vi "FindLineSubVI.vi"(0 "Image In":T1, 1 "Image Dst":T1, 7 "error in":errorcluster) -> (20 "Image Out":T1(plugin-control), 21 "Lines Calibrated (Shape Detection 1)":T2(array[cluster]) {"End Point"."Y" format="%.2f"; "End Point"."X" format="%.2f"; "Start Point"."Y" format="%.2f"; "Start Point"."X" format="%.2f"}, 27 "error out":errorcluster)   [LabVIEW 2011]
doc: "Creates, edits, and runs vision algorithms using NI Vision Assistant.\n\nWhen you place this Express VI on the block diagram, NI Vision Assistant launches. Create an algorithm using the Vision Assistant processing functions. After you create an algorithm, you can select the controls and indicators that you want to be able to programmatically set in LabVIEW. Double-click the Vision Assistant Express VI to edit the algorithm."
uses:
  <vilib>/vision/Image Controls.llb/IMAQ Image.ctl
  <vilib>/vision/NI_Vision_Development_Module.lvlib
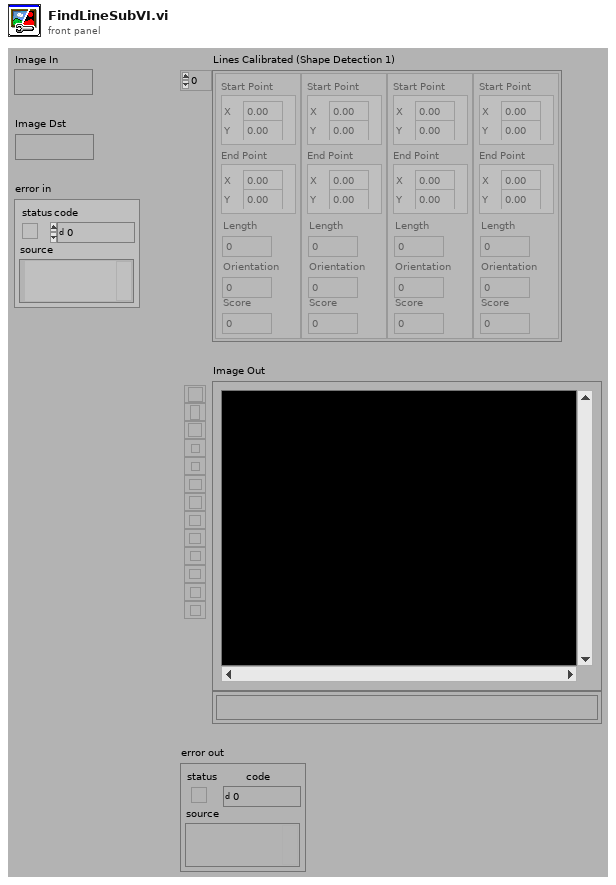
[diagram p1: front panel]
types:
  T1 = typedef "IMAQ Image.ctl" = refnum<image>
  T2 = cluster{"Start Point":cluster{"X":sgl, "Y":sgl}, "End Point":cluster{"X":sgl, "Y":sgl}, "Length":dbl, "Orientation":dbl, "Score":dbl}[]
  T3 = cluster{"Extraction Mode":u32, "Edge Threshold":i32, "Edge Filter Size":u32, "Min Length":i32, "Row Search Step Size":i32, "Col Search Step Size":i32, "Max Endpoint Gap":i32, "Closed":bool, "Subpixel":bool}
  T4 = cluster{"Rotation":bool, "Scale":bool, "Occlusion":bool, "Range Settings":cluster{"Match Constraints":u32, "Min":dbl, "Max":dbl}[]}
  T5 = cluster{"Global Rectangle":i32[], "Contours":cluster{"ID":enum32{"External", "Internal"}, "Type":u32, "Coordinates":i32[]}[]}
  T6 = typedef "Image Type" = u32
  T7 = cluster{"Start Point":cluster{"X":sgl, "Y":sgl}, "End Point":cluster{"X":sgl, "Y":sgl}, "Length":dbl, "Angle":dbl, "Score":dbl}[]
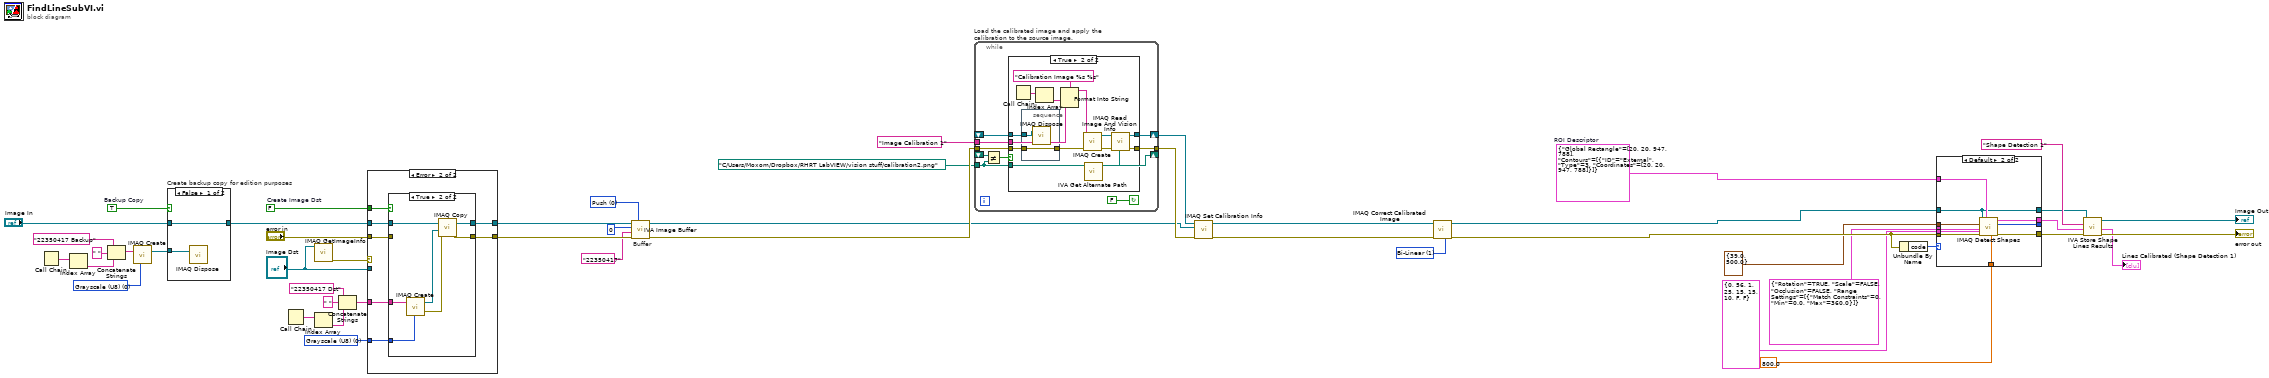
[diagram p0: block diagram]
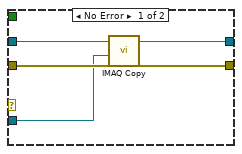
[diagram p4: hidden frame]
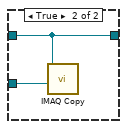
[diagram p6: hidden frame]
diagram:
  w10 = T5 {"Global Rectangle"=[20, 20, 947, 788], "Contours"=[{"ID"=enum."External", "Type"=3, "Coordinates"=[20, 20, 947, 788]}]}  # ROI Descriptor
  w17 = u32 1 items=["Zero Order", "Bi-Linear", "Quadratic", "Cubic Spline"] ("Interpolation Type")
  w26 = u16 0 items=["Push", "Pop", "Reset"] ("Function")
  w29 = T6 0 items=["Grayscale (U8)", "Grayscale (I16)", "Grayscale (SGL)", "Complex (CSG)", "RGB (U32)", "HSL (U32)", "RGB (U64)", "Grayscale (U16)"] ("Image Dst Type")
  w30 = T6 0 items=["Grayscale (U8)", "Grayscale (I16)", "Grayscale (SGL)", "Complex (CSG)", "RGB (U32)", "HSL (U32)", "RGB (U64)", "Grayscale (U16)"] ("Image Type")
  w49 = TRUE  # Backup Copy
  w42 = FALSE  # Create Image Dst
  # "Buffer"
  n1 = Call Chain() -> (call chain=w36:string[])
  n2 = Index Array(array=w36) -> (element=w35:string)  [unwired: 1 in]
  n3 = Concatenate Strings("22350417 Backup" ("Backup Image Name"), " ", w35) -> (w32:string)
  n4 = call "IMAQ Create"("Image Name"=w32, "Image Type"=w30) -> ("New Image"=w31:T1)  [unwired: 2 in, 2 out]
  n5 = case "Create backup copy for edition purposes" shown="False" w49 {
    tunnel: [w51 w53] -> w45
    tunnel: "Image In" -> [w51 w53]
    tunnel: w31 -> [w50 w52]
    frame False {
      n6 = call "IMAQ Dispose"("Image"=w50) -> ()  [unwired: 2 in, 4 out]
    }
    frame True {
      n7 = call "IMAQ Copy"("Image Dst"=w52, "Image Src"=w53) -> ()  [unwired: 1 in, 5 out]
    }
  }
  n8 = Call Chain() -> (call chain=w41:string[])
  n9 = call "IMAQ GetImageInfo"("Image"="Image Dst") -> ("error out"=w47:errorcluster)  [unwired: 1 in, 9 out]
  n10 = Index Array(array=w41) -> (element=w39:string)  [unwired: 1 in]
  n11 = Concatenate Strings("22350417 Dst" ("Image Dst Name"), " ", w39) -> (w37:string)
  n12 = case shown="Error" w47 {
    tunnel: [w58 w62] -> w28
    tunnel: [w57 w61] -> w43
    tunnel: w45 -> [w56 w63]
    tunnel: "error in" -> [w55 w59]
    tunnel: "Image Dst" -> [w54 _]
    tunnel: w37 -> [_ w65]
    tunnel: w29 -> [_ w64]
    tunnel: w42 -> [_ w60]
    frame No Error {
      n13 = call "IMAQ Copy"("error in (no error)"=w55, "Image Dst"=w54, "Image Src"=w56) -> ("error out"=w57:errorcluster, "Image Dst Out"=w58:T1)  [unwired: 3 out]
    }
    frame Error {
      n14 = case shown="True" w60 {
        tunnel: w65 -> [_ w74]
        tunnel: w64 -> [_ w73]
        tunnel: w63 -> [w67 w71]
        tunnel: [w67 w70] -> w62
        tunnel: [w66 w69] -> w61
        tunnel: w59 -> [w66 _]
        frame False {
        }
        frame True {
          n15 = call "IMAQ Create"("Image Name"=w74, "Image Type"=w73) -> ("New Image"=w72:T1, "error out"=w68:errorcluster)  [unwired: 2 in, 1 out]
          n16 = call "IMAQ Copy"("error in (no error)"=w68, "Image Dst"=w72, "Image Src"=w71) -> ("error out"=w69:errorcluster, "Image Dst Out"=w70:T1)  [unwired: 3 out]
        }
      }
    }
  }
  n17 = call <vilib>:"IVA Image Buffer.vi"("Function"=w26, "error in (no error)"=w43, "Prefix"="22350417", "Buffer #"=0, "Image In"=w28) -> ("error out"=w27:errorcluster, "Image Out"=w19:T1)  [unwired: 5 out]
  n18 = while "Load the calibrated image and apply the calibration to the source image." {
    shift-right: [w83] -> w22
    shift-left: _ -> [w82]
    tunnel: [w80] -> w21
    tunnel: w27 -> [w79]
    tunnel: path "C:/Users/Moxom/Dropbox/RHRT LabVIEW/vision stuff/calibration2.png" ("File Path") -> [w75]
    tunnel: "Image Calibration 1" ("Step Name") -> [w78]
    shift-right: [w75] -> _
    shift-left: _ -> [w77]
    stop <- FALSE continue-if-true
    n19 = Not Equal?(x=w77, y=w75) -> (x != y?=w76:bool)
    n20 = case shown="True" w76 {
      tunnel: [w85 w97] -> w83
      tunnel: w82 -> [w85 w89]
      tunnel: [w84 w94] -> w80
      tunnel: w79 -> [w84 w90]
      tunnel: w75 -> [_ w87]
      tunnel: w78 -> [_ w91]
      frame False {
      }
      frame True {
        n21 = Call Chain() -> (call chain=w93:string[])
        n22 = stacked-sequence {
          tunnel: w90 -> [w100]
          tunnel: w89 -> [w101]
          tunnel: [w100] -> w88
          frame #0 {
            n23 = call "IMAQ Dispose"("Image"=w101) -> ()  [unwired: 2 in, 4 out]
          }
        }
        n24 = Index Array(array=w93) -> (element=w92:string)  [unwired: 1 in]
        n25 = Format Into String(format string="Calibration Image %s %s" ("Image Name"), w92, w91) -> (resulting string=w99:string)  [unwired: 2 in, 1 out]
        n26 = call "IMAQ Create"("Image Name"=w99, "error in (no error)"=w88) -> ("New Image"=w96:T1, "error out"=w95:errorcluster)  [unwired: 2 in, 1 out]
        n27 = call <vilib>:"IVA Get Alternate Path.vi"("Path In"=w87) -> ("Path Out"=w86:path)  [unwired: 10 out]
        n28 = call "IMAQ Read Image And Vision Info"("File Path"=w86, "error in (no error)"=w95, "Image"=w96) -> ("error out"=w94:errorcluster, "Image Out"=w97:T1)  [unwired: 1 in, 6 out]
      }
    }
  }
  n29 = call "IMAQ Set Calibration Info"("error in (no error)"=w21, "Image Dst"=w19, "Image Src"=w22) -> ("error out"=w20:errorcluster, "Calibrated Image"=w15:T1)  [unwired: 1 in, 6 out]
  n30 = call "IMAQ Correct Calibrated Image"("Interpolation Type"=w17, "error in (no error)"=w20, "Image Src"=w15) -> ("error out"=w16:errorcluster, "Corrected Image"=w9:T1)  [unwired: 4 in, 3 out]
  n31 = Unbundle By Name(w16) -> ("code"=w3:i32)
  n32 = case shown="Default" w3 {
    tunnel: w16 -> [_ w112]
    tunnel: [_ w111] -> _
    tunnel: T4 {"Rotation"=TRUE, "Scale"=FALSE, "Occlusion"=FALSE, "Range Settings"=[{"Match Constraints"=0, "Min"=0.0, "Max"=360.0}]} ("Match Options") -> [_ w110]
    tunnel: T3 {"Extraction Mode"=0, "Edge Threshold"=56, "Edge Filter Size"=1, "Min Length"=25, "Row Search Step Size"=15, "Col Search Step Size"=15, "Max Endpoint Gap"=10, "Closed"=FALSE, "Subpixel"=FALSE} ("Curve Parameters") -> [_ w109]
    tunnel: 800.0 ("Minimum match score") -> [_ w108]
    tunnel: cluster{"Min Radius":dbl, "Max Radius":dbl} {"Min Radius"=39.0, "Max Radius"=500.0} ("Line Descriptor") -> [_ w107]
    tunnel: w10 -> [_ w106]
    tunnel: w9 -> [w102 w103]
    tunnel: [_ w105] -> w7
    tunnel: [_ w104] -> w6
    tunnel: [w102 w103] -> w2
    frame -1074396199, -1074396198 {
      # "Discard Coordinate\nSystem Error"
    }
    frame Default {
      n33 = call-poly "IMAQ Detect Shapes"("Minimum match score"=w108, "Curve Parameters"=w109, "ROI Descriptor"=w106, "error in (no error)"=w112, "Match Options"=w110, "Line Descriptor"=w107, "Image"=w103) -> ("error out"=w104:errorcluster, "Number of Matches Returned"=w111:i32, "Lines"=w105:T7)  [unwired: 2 out]
    }
  }
  n34 = call <vilib>:"IVA Store Shape Lines Results.vi"("error in (no error)"=w6, "Lines"=w7, "Step Name"="Shape Detection 1", "Image in"=w2) -> ("error out"=→"error out":errorcluster, "Lines Calibrated"=→"Lines Calibrated (Shape Detection 1)":T2, "Image dup"=→"Image Out":T1)  [unwired: 5 out]
